vi "scan_continuous_helper.vi"(8 "error in (no error)":errorcluster, 9 "scan_desc":T2, 10 "chav":T1[](array[typedef]), 11 "DAQ ID":string="usbbase") -> (0 "error out":errorcluster, 1 "scan_desc out":T2, 2 "chav out":T1[](array[typedef]), 3 "data":sgl[](array[numeric]))   [LabVIEW 2021, in "libad4.lvlib"]
doc: "Helper function to perform continuous DAQ scan."
uses:
  <userlib>/libad4/libad4.lvlib
  <userlib>/libad4/controls/ad scan cha desc.ctl
  <userlib>/libad4/controls/ad scan desc.ctl
  <userlib>/libad4/controls/ad scan state.ctl
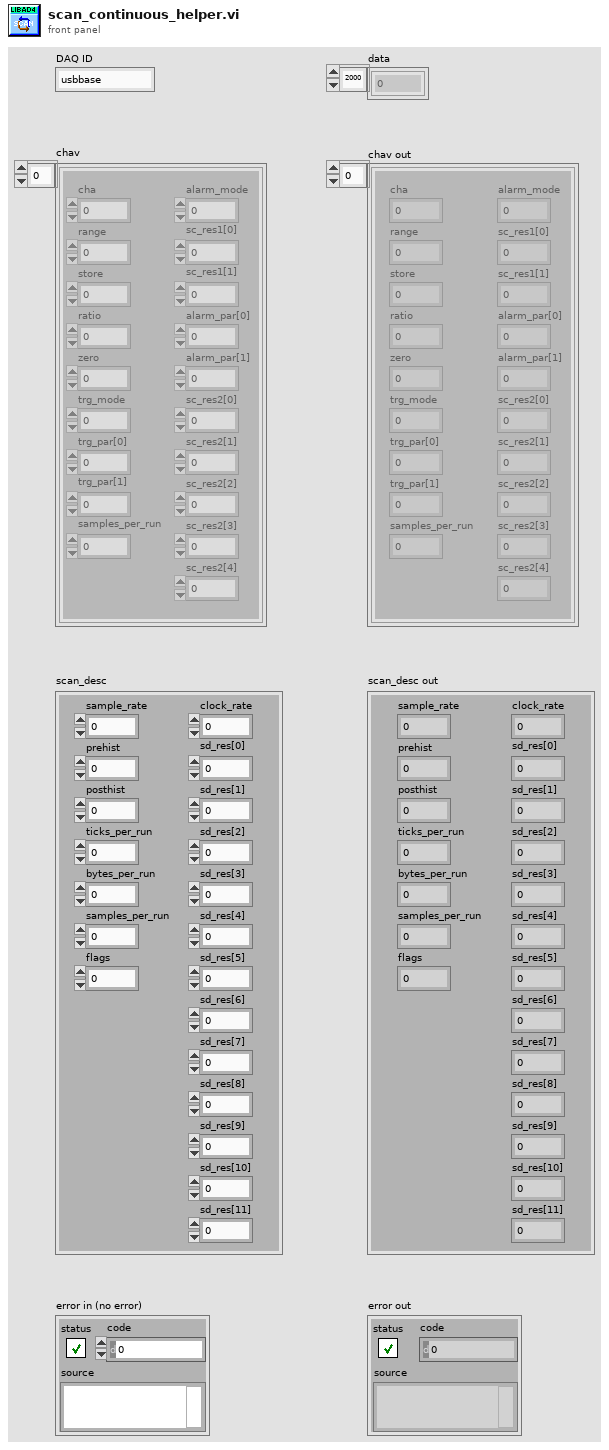
[diagram p1: front panel]
types:
  T1 = typedef "libad4.lvlib/ad scan cha desc.ctl" = cluster{"cha":i32, "range":i32, "store":i32, "ratio":i32, "zero":u32, "trg_mode":u8, "alarm_mode":u8, "sc_res1[0]":u8, "sc_res1[1]":u8, "trg_par[0]":u32, "trg_par[1]":u32, "samples_per_run":i32, "alarm_par[0]":u32, "alarm_par[1]":u32, "sc_res2[0]":u32, "sc_res2[1]":u32, "sc_res2[2]":u32, "sc_res2[3]":u32, "sc_res2[4]":u32}
  T2 = typedef "libad4.lvlib/ad scan desc.ctl" = cluster{"sample_rate":dbl, "clock_rate":dbl, "prehist":u64, "posthist":u64, "ticks_per_run":u32, "bytes_per_run":u32, "samples_per_run":u32, "flags":u32, "sd_res[0]":u32, "sd_res[1]":u32, "sd_res[2]":u32, "sd_res[3]":u32, "sd_res[4]":u32, "sd_res[5]":u32, "sd_res[6]":u32, "sd_res[7]":u32, "sd_res[8]":u32, "sd_res[9]":u32, "sd_res[10]":u32, "sd_res[11]":u32}
  T3 = typedef "libad4.lvlib/ad scan state.ctl" = cluster{"flags":i32, "runs_pending":i32, "posthist":i64}
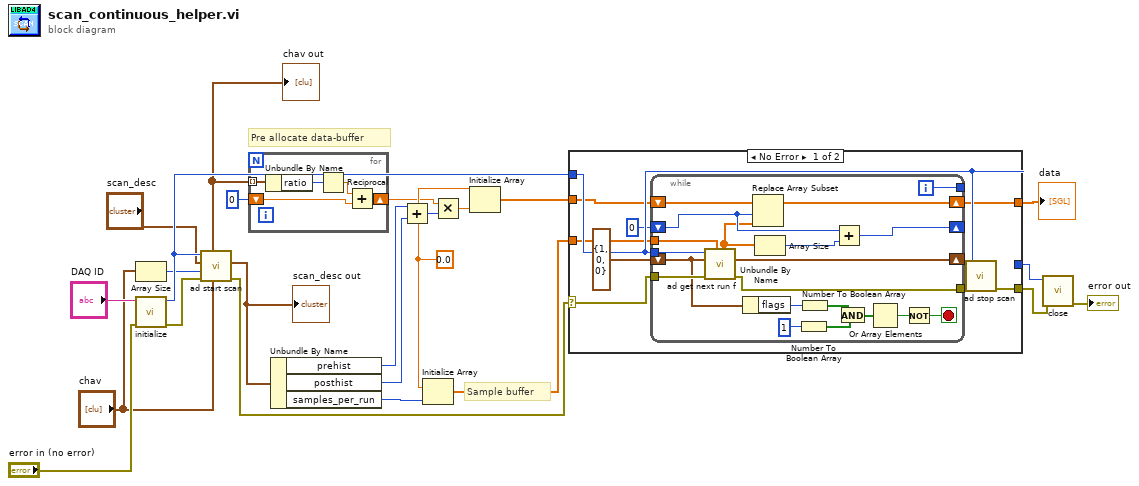
[diagram p0: block diagram]
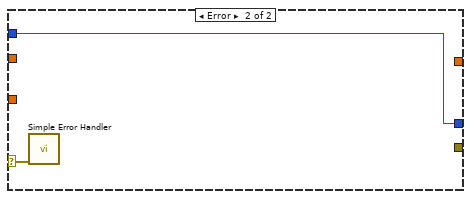
[diagram p2: hidden frame]
diagram:
  w10 = sgl 0.0 ("element")
  # "Pre allocate data-buffer"
  # "Sample buffer"
  n1 = Array Size(array="chav") -> (size(s)=w14:i32)
  n2 = call <userlib>:"initialize.vi"("error in (no error)"="error in (no error)", "name"="DAQ ID") -> ("error out"=w20:errorcluster, "function return"=w23:i32)  [unwired: 8 in]
  n3 = call <userlib>:"ad start scan.vi"("chav"="chav", "error in (no error)"=w20, "chac"=w14, "scan_desc"="scan_desc", "adh"=w23) -> ("error out"=w18:errorcluster, "scan_desc out"=w13:T2, "chav out"=w6:T1[])  [unwired: 3 in, 1 out]
  "scan_desc out" <- w13
  "chav out" <- w6
  n4 = for {
    tunnel: w6 -> [w29] mode=indexing
    shift-right: [w25] -> w2
    shift-left: 0 -> [w26]
    n5 = Unbundle By Name(w29) -> ("ratio"=w28:i32)
    n6 = Reciprocal(x=w28) -> (1/x=w27:dbl)
    n7 = Add(x=w27, y=w26) -> (x+y=w25:dbl)
  }
  n8 = Unbundle By Name(w13) -> ("prehist"=w9:u64, "posthist"=w8:u64, "samples_per_run"=w11:u32)
  n9 = Add(x=w9, y=w8) -> (x+y=w4:u64)
  n10 = Initialize Array(w10, w11) -> (w12:sgl[])
  n11 = Multiply(x=w2, y=w4) -> (x*y=w5:dbl)
  n12 = Initialize Array(w10, w5) -> (w7:sgl[])
  n13 = case shown="No Error" w18 {
    selector: w18 -> [w37 w59]
    tunnel: w23 -> [w36 w60]
    tunnel: [w38 _] -> w21
    tunnel: [w36 w60] -> w24
    tunnel: [w32 _] -> w1
    tunnel: w12 -> [w33 _]
    tunnel: w7 -> [w30 _]
    frame No Error {
      n14 = while {
        tunnel: w37 -> [w58]
        tunnel: w36 -> [w57]
        tunnel: [w56] -> w35
        shift-right: [w53] -> w32
        shift-left: w30 -> [w52]
        shift-right: [w55] -> _
        shift-left: 0 ("disabled index (col)") -> [w51]
        tunnel: w33 -> [w54]
        shift-right: [w48] -> _
        shift-left: T3 {"flags"=1, "runs_pending"=0, "posthist"=0} ("state out") -> [w47]
        tunnel: [w39] -> _
        i -> [w39]
        stop <- w40 stop-if-true
        n15 = call <userlib>:"ad get next run f.vi"("buffer"=w54, "error in (no error)"=w58, "state"=w47, "adh"=w57) -> ("error out"=w56:errorcluster, "state out"=w48:T3, "buffer out"=w49:sgl[])  [unwired: 3 in, 2 out]
        n16 = Unbundle By Name(w47) -> ("flags"=w46:i32)
        n17 = Replace Array Subset(array=w52, new element=w49, index=w51) -> (w53:sgl[])
        n18 = Array Size(array=w49) -> (size(s)=w50:i32)
        n19 = Number To Boolean Array(number=1) -> (Boolean array=w43:bool[])
        n20 = Number To Boolean Array(number=w46) -> (Boolean array=w45:bool[])
        n21 = Add(x=w51, y=w50) -> (x+y=w55:i32)
        n22 = And(x=w45, y=w43) -> (x .and. y?=w44:bool[])
        n23 = Or Array Elements(Boolean array=w44) -> (logical OR=w41:bool)
        n24 = Not(x=w41) -> (.not. x?=w40:bool)
      }
      n25 = call <userlib>:"ad stop scan.vi"("error in (no error)"=w35, "adh"=w36) -> ("error out"=w38:errorcluster)  [unwired: 7 in, 2 out]
    }
    frame Error {
      n26 = call <vilib>:"Simple Error Handler.vi"("error in (no error)"=w59) -> ()  [unwired: 4 in, 5 out]
    }
  }
  "data" <- w1
  n27 = call <userlib>:"close.vi"("error in (no error)"=w21, "adh"=w24) -> ("error out"=→"error out":errorcluster)  [unwired: 8 in, 1 out]
